vi "Configure Average.vi"(7 "Average on":bool, 8 "error in (no error)":errorcluster, 10 "Average Count":i32, 11 "PM-EMP in":refnum<class "PM-EMP.lvclass">) -> (0 "error out":errorcluster, 3 "PM-EMP out":refnum<class "PM-EMP.lvclass">)   [LabVIEW 2020, in "PM-EMP.lvclass"]
uses:
  PM-EMP.lvclass
  C:/Sandbox/Git_Sandbox/WiSpry Test Framework source code (LV20)/WiSpry Test Framework/Instruments/Instrument.lvclass
  C:/Sandbox/Git_Sandbox/WiSpry Test Framework source code (LV20)/WiSpry Test Framework/Instruments/Power Meter/Power Meter.lvclass
  Instrument.lvclass/Instrument.ctl
  Power Meter.lvclass/Power Meter.ctl
  Instrument.lvclass
  Power Meter.lvclass
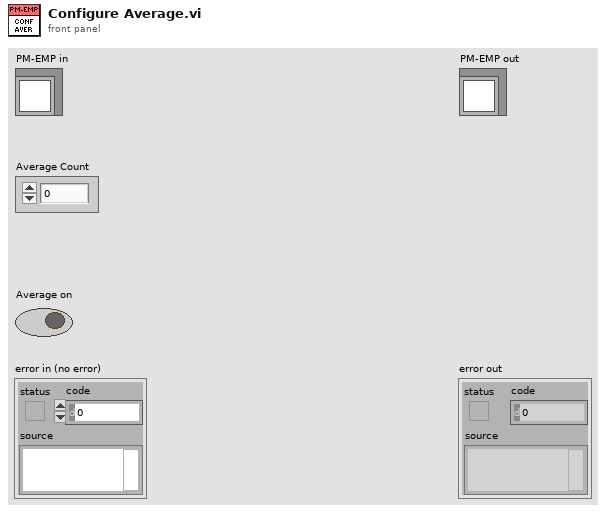
[diagram p1: front panel]
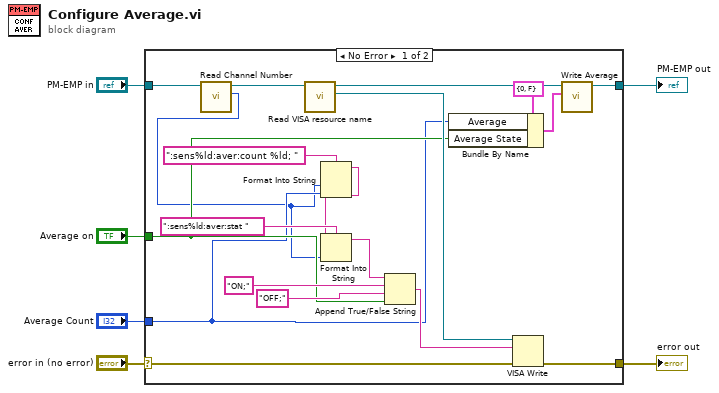
[diagram p0: block diagram]
diagram:
  n1 = case shown="No Error" "error in (no error)" {
    selector: "error in (no error)" -> [w24 w27]
    tunnel: "PM-EMP in" -> [w9 w26]
    tunnel: [w23 w27] -> w4
    tunnel: "Average on" -> [w14 _]
    tunnel: "Average Count" -> [w10 _]
    tunnel: [w21 w26] -> w1
    frame No Error {
      n2 = call-dynamic "Read Channel Number.vi"("Power Meter in"=w9) -> ("Channel Number"=w7:u8, "Power Meter out"=w8:refnum<class "PM-EMP.lvclass">)  [unwired: 9 in]
      n3 = call "Read VISA resource name.vi"("Instrument in"=w8) -> ("VISA resource name"=w25:refnum<visa-resource-name>, "Instrument out"=w22:refnum<class "PM-EMP.lvclass">)  [unwired: 9 in]
      n4 = Format Into String(format string=":sens%ld:aver:count %ld; " ("string (\"\")"), w7, w10) -> (resulting string=w12:string)  [unwired: 2 in, 1 out]
      n5 = Format Into String(format string=":sens%ld:aver:stat " ("string (\"\")"), initial string=w12, w7) -> (resulting string=w18:string)  [unwired: 1 in, 1 out]
      n6 = Append True/False String(1:w14, 2:"OFF;" ("false string"), 3:"ON;" ("true string"), 4:w18) -> (0:w11:string)
      n7 = Bundle By Name(cluster=cluster{"Average":i32, "Average State":bool} {"Average"=0, "Average State"=FALSE} ("Average"), "Average"=w10, "Average State"=w14) -> (w19:cluster{"Average":i32, "Average State":bool})
      n8 = VISA Write(VISA resource name=w25, write buffer=w11, error in (no error)=w24) -> (error out=w23:errorcluster)  [unwired: 2 out]
      n9 = call "Write Average.vi"("Average"=w19, "Power Meter in"=w22) -> ("Power Meter out"=w21:refnum<class "PM-EMP.lvclass">)  [unwired: 9 in]
    }
    frame Error {
    }
  }
  "error out" <- w4
  "PM-EMP out" <- w1
